vi "Get Channel Names and Default Values.vi"(8 "error in":errorcluster, 10 "channels":refnum<class "Channel.lvclass">[](array[class]), 11 "PWM mode in":refnum<class "PWM Mode.lvclass">) -> (0 "error out":errorcluster, 1 "default values":dbl[](array[numeric]), 2 "names":string[](array[string]), 3 "PWM mode out":refnum<class "PWM Mode.lvclass">)   [LabVIEW 2017, in "Scan Engine Scripting.lvlib" / "PWM Mode.lvclass"]
uses:
  PWM Mode.lvclass
  Channel Classes/Channel/Channel.lvclass
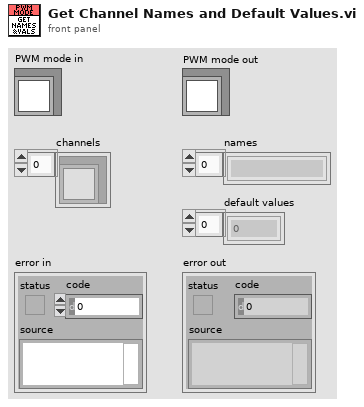
[diagram p1: front panel]
types:
  T1 = typedef "Scan Engine Scripting.lvlib/pwm channel settings.ctl" = cluster{"name":string, "default value":dbl, "frequency":T2}
  T2 = typedef "Scan Engine Scripting.lvlib/PWM Output Channel.lvclass/Frequency.ctl" = enum16{"1 Hz (1,000,000 us)", "50 Hz (20,000 us)", "250 Hz (4,000 us)", "500 Hz (2,000 us)", "1 kHz (1,000 us)", "5 kHz (200 us)", "10 kHz (100 us)", "20 kHz (50 us)"}
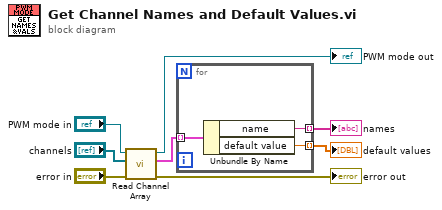
[diagram p0: block diagram]
diagram:
  n1 = call "Read Channel Array.vi"("error in"="error in", "channels"="channels", "digital output mode in"="PWM mode in") -> ("error out"=→"error out":errorcluster, "channel settings"=w4:T1[], "digital output mode out"=→"PWM mode out":refnum<class "PWM Mode.lvclass">)  [unwired: 6 in]
  n2 = for {
    tunnel: w4 -> [w11] mode=indexing
    tunnel: [w9] -> w3 mode=indexing
    tunnel: [w10] -> w2 mode=indexing
    n3 = Unbundle By Name(w11) -> ("name"=w9:string, "default value"=w10:dbl)
  }
  "names" <- w3
  "default values" <- w2
